vi "Sensor Scaling.vi"(8 "error in":errorcluster) -> (0 "error out":errorcluster, 3 "Output":cluster{"X":dbl[], "Y":dbl[], "Avg point":i16}[](array[cluster]))   [LabVIEW 2015]
uses:
  <vilib>/Analysis/NI_AALPro.lvlib
panel:
  in  "Avg Point":i16=1 min=1 max=500
  out "Offset":dbl format="%0.2f"
  out "Slope":dbl format="%0.2f"
  in  "Unit":string
  in  "Sensor":u16(ring) items=["Load Cell", "LVDT", "LOadcell1", "wq", "load3", "LVDT3", "gggh"]
  in  "Next":bool
  in  "Input Values":dbl[](array[numeric])
  in  "New Calibration":dbl[](array[numeric])
  in  "Sensor Add":bool
  in  "Graph Plot":bool
  in  "Help Button":bool
  in  "Quit":bool
  in  "Save":bool
  out "XY Graph":T1(graph)
  out "error out 2":errorcluster
  out "Numeric":dbl
  out "Old Calibration":dbl[](array[numeric])
  # "Sensor Calibration"
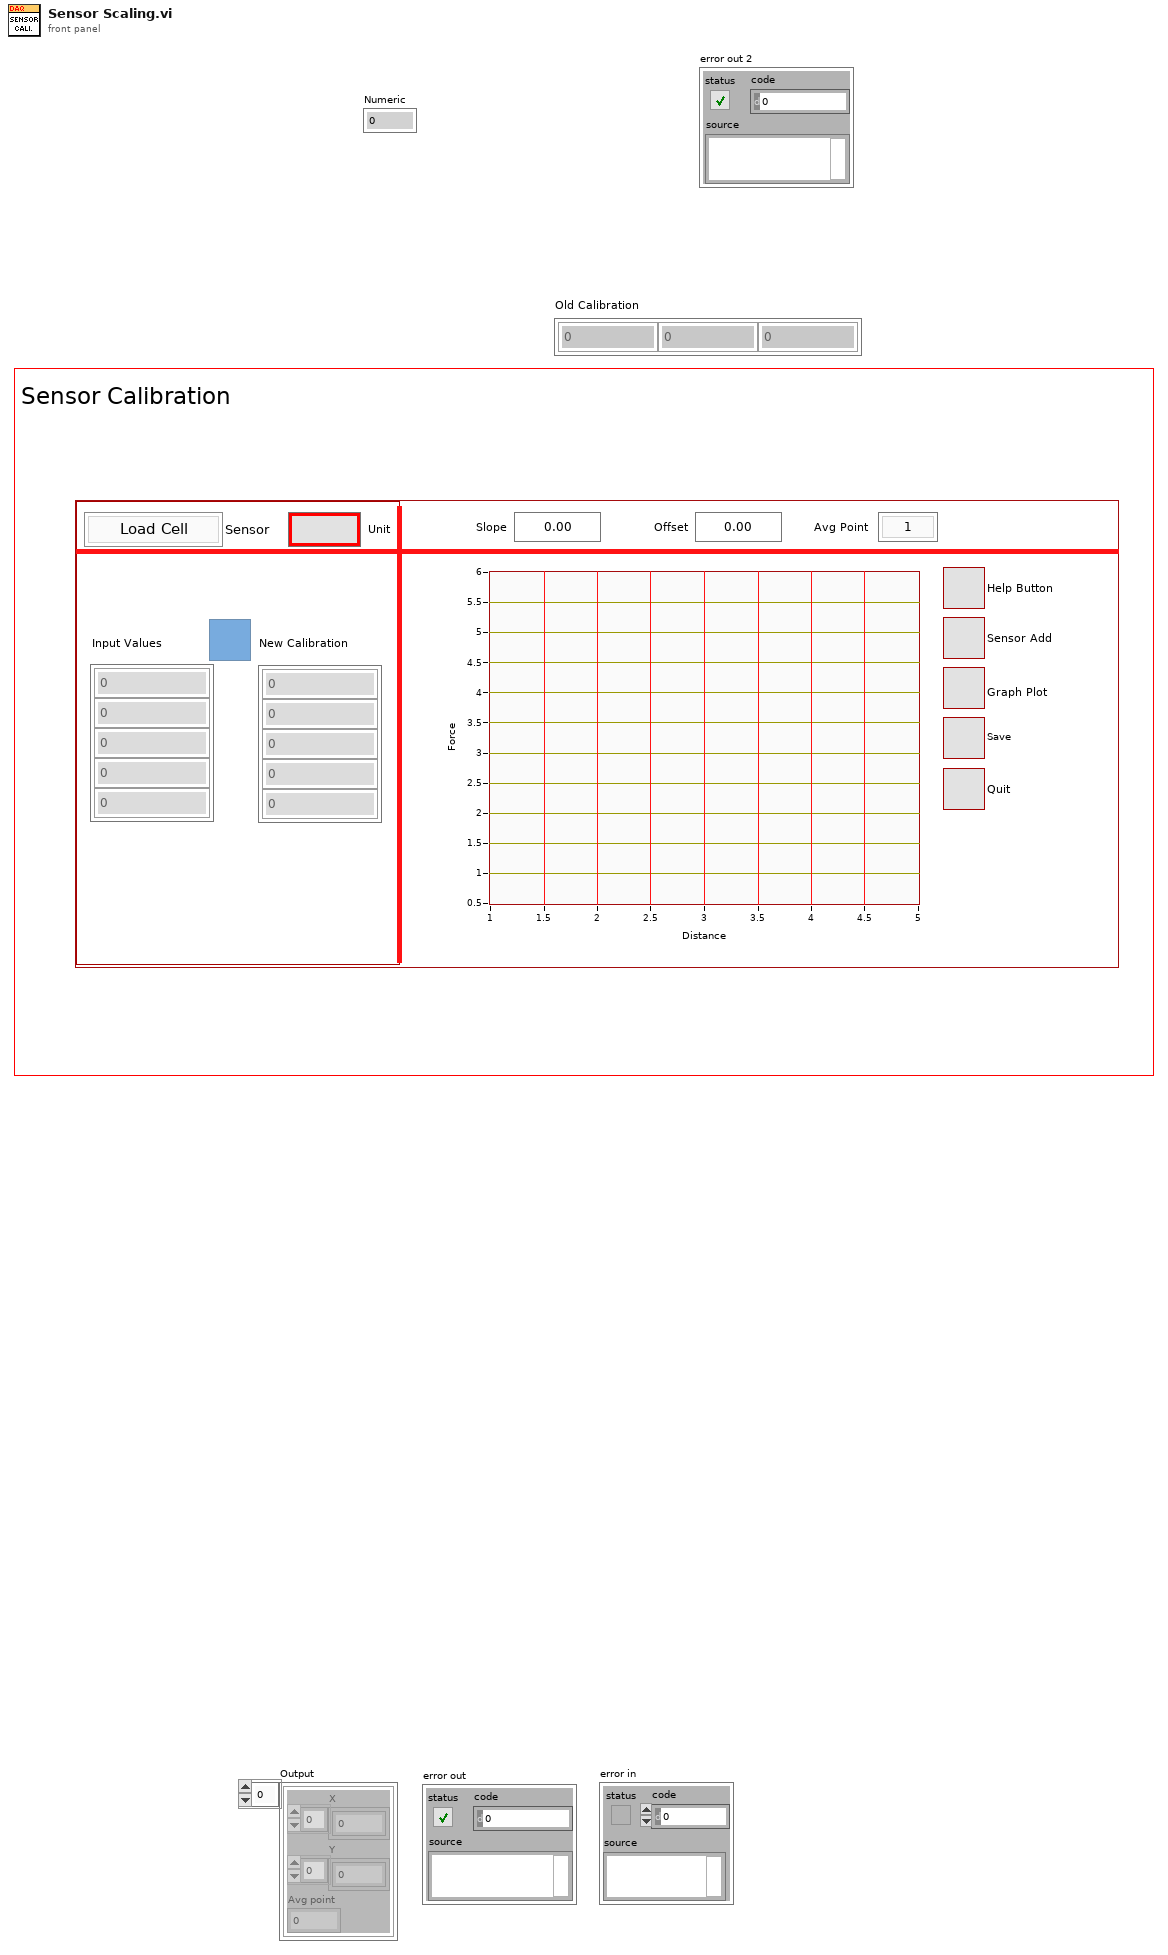
[diagram p1: front panel]
types:
  T1 = cluster{"Input Values":dbl[], "New Calibration":dbl[]}
  T2 = cluster{"XInput":dbl[], "Y New Value":dbl[], "Avg point":i16}[]
  T3 = cluster{"XInput":dbl[], "Y New Value":dbl[], "Avg point":i16}
  T4 = cluster{"Input Values":dbl[], "New Calibration":dbl[], "Sensor":u16}
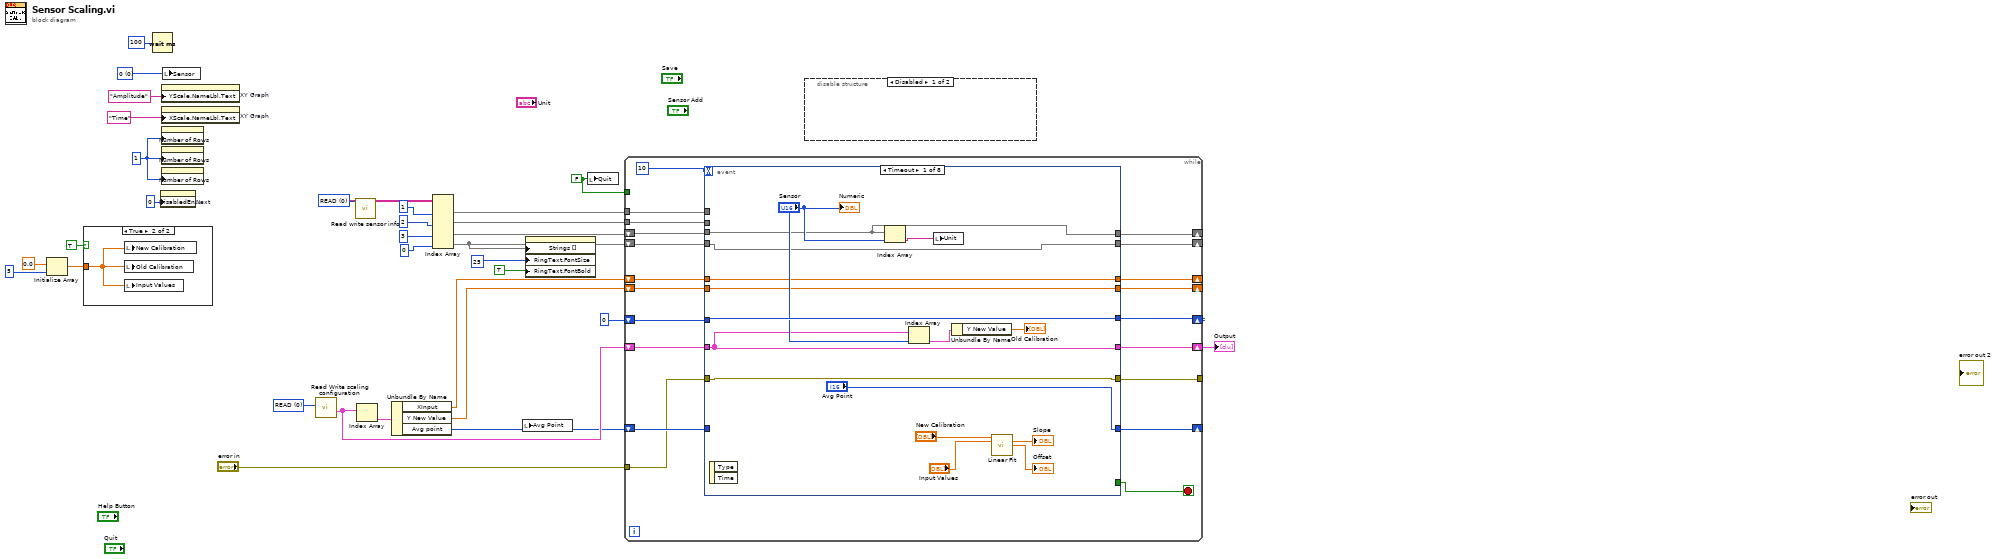
[diagram p0: block diagram]
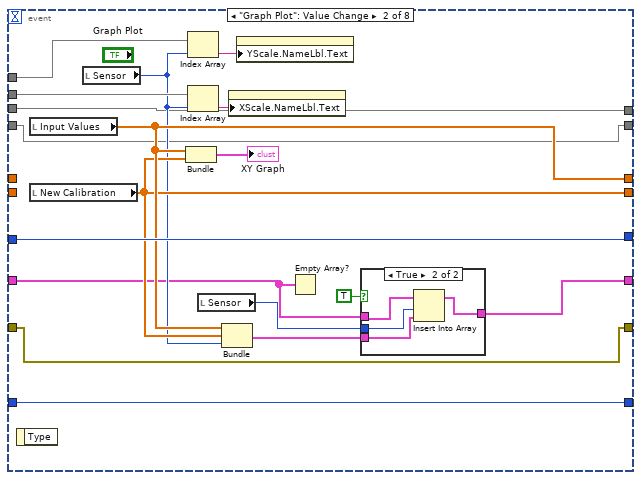
[diagram p4: hidden frame]
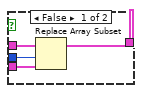
[diagram p5: hidden frame]
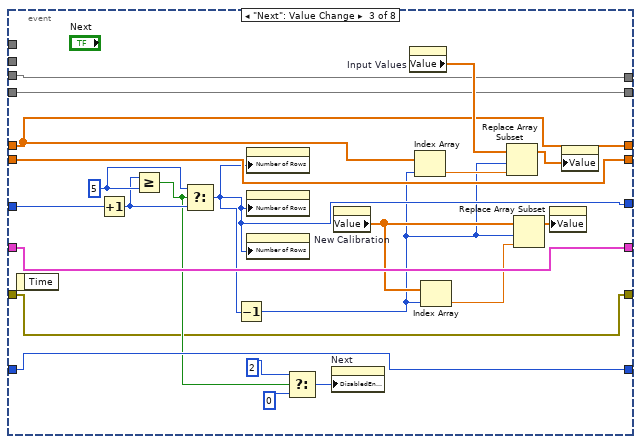
[diagram p6: hidden frame]
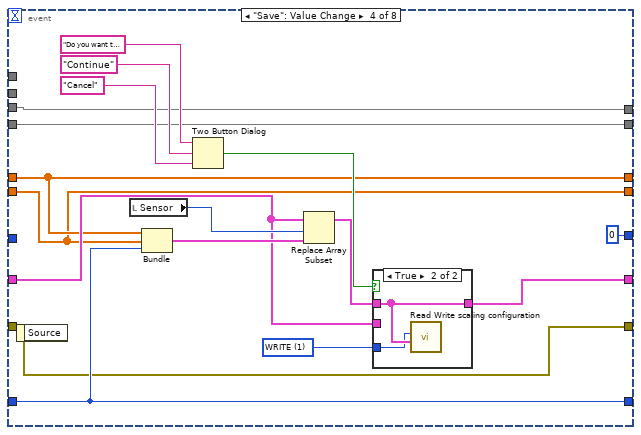
[diagram p7: hidden frame]
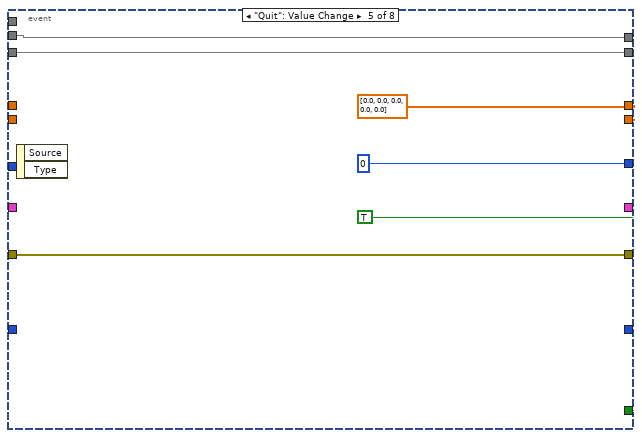
[diagram p9: hidden frame]
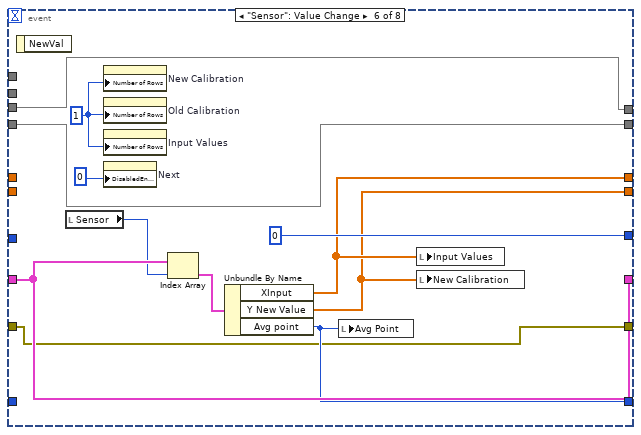
[diagram p10: hidden frame]
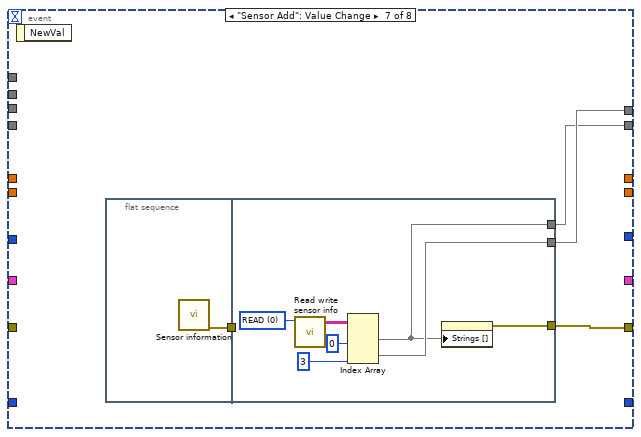
[diagram p11: hidden frame]
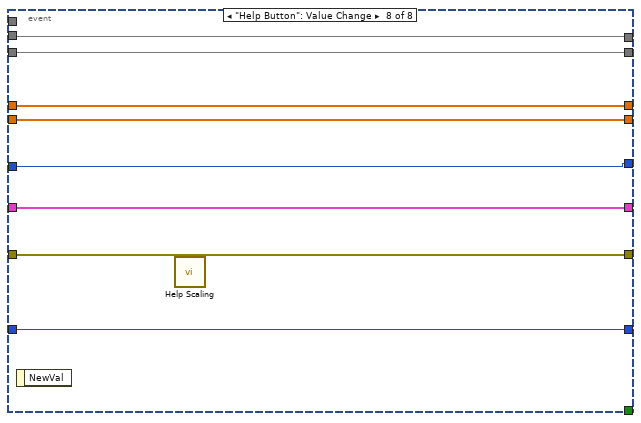
[diagram p12: hidden frame]
diagram:
  w3 = FALSE ("Quit")
  w13 = u16 0 items=["READ", "WRITE"] ("Read/Write")
  w21 = u16 0 items=["READ", "WRITE"] ("Read/Write")
  w9 = u32 1 ("Number of Rows")
  w29 = u16 0 items=["0", "1", "2", "3", "4", "5", "6", "7", "8", "9", "10", "11", "12", "13", "14", "15", "16", "17", "18", "19", "20", "21", "22", "23", "24", "25", "26", "27", "28", "29"] ("Ring")
  n1 = Initialize Array(0.0 ("element"), 5 ("dimension size")) -> (w20:dbl[])
  n2 = case shown="True" TRUE {
    tunnel: w20 -> [_ w33]
    frame False {
    }
    frame True {
      n3 = local write "New Calibration"(w33) -> ()
      n4 = local write "Old Calibration"(w33) -> ()
      n5 = local write "Input Values"(w33) -> ()
    }
  }
  n6 = Wait (ms)(milliseconds to wait=u32 100) -> ()  [unwired: 1 out]
  n7 = property on="Next" class="Bool"("DisabledEnum"=u16 0) -> ()  [unwired: 2 in, 2 out]
  n8 = property on="XY Graph" class="XYGraph (strict)"("YScale.NameLbl.Text"="Amplitude" ("Y Scale.Name Label.Text")) -> ()  [unwired: 2 in, 2 out]
  n9 = property on="XY Graph" class="XYGraph (strict)"("XScale.NameLbl.Text"="Time" ("X Scale.Unit Label.Text")) -> ()  [unwired: 2 in, 2 out]
  n10 = property on="Old Calibration" class="Arr (strict)"("Number of Rows"=w9) -> ()  [unwired: 2 in, 2 out]
  n11 = property on="Input Values" class="Arr (strict)"("Number of Rows"=w9) -> ()  [unwired: 2 in, 2 out]
  n12 = property on="New Calibration" class="Arr (strict)"("Number of Rows"=w9) -> ()  [unwired: 2 in, 2 out]
  n13 = local write "Sensor"(w29) -> ()
  n14 = call "Read Write scaling configuration.vi"("Read/Write"=w21) -> ("Output"=w18:T2)  [unwired: 4 in, 2 out]
  n15 = call "Read write sensor info.vi"("Read/Write"=w13) -> ("Table Control out"=w12:string[][])  [unwired: 9 in, 1 out]
  n16 = Index Array(array=w18) -> (element=w19:T3)  [unwired: 1 in]
  n17 = Unbundle By Name(w19) -> ("XInput"=w7:dbl[], "Y New Value"=w6:dbl[], "Avg point"=w16:i16)
  n18 = Index Array(array=w12, index (col) #1=1 ("disabled index (col)"), index (col) #2=2 ("index (row)"), index (col) #3=3 ("index (row)"), index (col) #4=0 ("index (row)")) -> (element #1=w26:string[], element #2=w25:string[], element #3=w5:string[], element #4=w4:string[])  [unwired: 4 in]
  n19 = local write "Avg Point"(w16) -> ()
  n20 = property on="Sensor" class="Ring (strict)"("Strings []"=w4, "RingText.FontSize"=u32 25 ("Ring Text.Font:Size"), "RingText.FontBold"=TRUE ("Ring Text.Font:Bold")) -> ()  [unwired: 2 in, 2 out]
  n21 = local write "Quit"(w3) -> ()
  n22 = while {
    shift-right: [w51] -> _
    shift-left: i8 0 -> [w52]
    shift-right: [w50] -> _
    shift-left: w6 -> [w49]
    tunnel: w26 -> [w47]
    tunnel: w25 -> [w46]
    shift-right: [w45] -> _
    shift-left: w7 -> [w44]
    shift-right: [w42] -> w15
    shift-left: w18 -> [w43]
    shift-right: [w41] -> _
    shift-left: w16 -> [w40]
    tunnel: [w38] -> _
    tunnel: "error in" -> [w35]
    shift-right: [w37] -> _
    shift-left: w5 -> [w36]
    shift-right: [w34] -> _
    shift-left: w4 -> [w39]
    tunnel: w3 -> [_]
    stop <- w48 stop-if-true
    n23 = event shown="[0] Timeout" {
      selector: _ -> [_ _ _ _ _ _ _ _]
      dyn-events: _ -> [_ _ _ _ _ _ _ _]
      timeout: 10 -> [_ _ _ _ _ _ _ _]
      tunnel: [_ _ _ _ TRUE _ _ _] -> w48
      tunnel: w52 -> [w69 w83 w117 _ _ _ _ w170]
      tunnel: [w69 w83 w107 i8 0 i8 0 i8 0 ("y") _ w170] -> w51
      tunnel: [w63 w77 w113 w122 w141 w147 _ w173] -> w50
      tunnel: w49 -> [w63 _ w113 w122 _ _ _ w173]
      tunnel: w47 -> [_ w87 _ _ _ _ _ _]
      tunnel: w46 -> [_ w86 _ _ _ _ _ _]
      tunnel: w36 -> [w57 w72 w98 w120 w140 w146 _ w175]
      tunnel: [w64 w78 w110 w123 w141 w148 _ w174] -> w45
      tunnel: w44 -> [w64 _ w110 w123 _ _ _ w174]
      tunnel: w43 -> [w65 w74 w114 w125 _ w154 _ w172]
      tunnel: [w65 w75 w114 w129 _ w154 _ w172] -> w42
      tunnel: ["Avg Point" w82 w106 w126 _ w151 _ w171] -> w41
      tunnel: w40 -> [_ w82 w106 w126 _ _ _ w171]
      tunnel: w39 -> [w55 w70 w96 w118 w138 w144 _ w168]
      tunnel: [w56 w71 w97 w119 w139 w145 w158 w169] -> w38
      tunnel: [w57 w72 w98 w120 w140 w146 w157 w175] -> w37
      tunnel: w35 -> [w56 w71 w97 w119 w139 w145 _ w169]
      tunnel: [w55 w70 w96 w118 w138 w144 w156 w168] -> w34
      event Timeout {
        n24 = event-data() -> ()  [unwired: 3 out]
        n25 = Index Array(array=w57, index="Sensor") -> (element=w54:string)
        n26 = Index Array(array=w65, index="Sensor") -> (element=w67:T3)
        n27 = local write "Unit"(w54) -> ()
        n28 = Unbundle By Name(w67) -> ("Y New Value"=→"Old Calibration":dbl[])
        n29 = call <vilib>:"Linear Fit.vi"("Y"="New Calibration", "X"="Input Values") -> ("slope"=→"Slope":dbl, "intercept"=→"Offset":dbl)  [unwired: 9 in, 3 out]
        "Numeric" <- "Sensor"
      }
      event "Graph Plot": Value Change {
        n30 = event-data() -> ()  [unwired: 2 out]
        n31 = local read "Input Values"() -> (w78:dbl[])
        n32 = local read "New Calibration"() -> (w77:dbl[])
        n33 = local read "Sensor"() -> (w76:u16)
        n34 = Bundle("Input Values"=w78, "New Calibration"=w77) -> (→"XY Graph":T1)  [unwired: 1 in]
        n35 = Index Array(array=w87, index=w76) -> (element=w85:string)
        n36 = Index Array(array=w86, index=w76) -> (element=w84:string)
        n37 = local read "Sensor"() -> (w79:u16)
        n38 = Bundle("Input Values"=w78, "New Calibration"=w77, "Sensor"=w76) -> (w80:T4)  [unwired: 1 in]
        n39 = property on="XY Graph" class="XYGraph (strict)"("XScale.NameLbl.Text"=w84) -> ()  [unwired: 2 in, 2 out]
        n40 = property on="XY Graph" class="XYGraph (strict)"("YScale.NameLbl.Text"=w85) -> ()  [unwired: 2 in, 2 out]
        n41 = Empty Array?(array=w74) -> ()  [unwired: 1 out]
        n42 = case shown="True" TRUE {
          tunnel: w80 -> [w91 w93]
          tunnel: w79 -> [w90 w95]
          tunnel: w74 -> [w89 w94]
          tunnel: [w88 w92] -> w75
          frame False {
            n43 = Replace Array Subset(array=w89, new element=w91, index=w90) -> (w88:T2)
          }
          frame True {
            n44 = Insert Into Array(array=w94, index=w95, new element=w93) -> (w92:T2)
          }
        }
      }
      event "Next": Value Change {
        w116 = i8 5 ("y")
        n45 = event-data() -> ()  [unwired: 2 out]
        n46 = Increment(x=w117) -> (x+1=w115:i8)
        n47 = Greater Or Equal?(x=w115, y=w116) -> (x >= y?=w105:bool)
        n48 = Select(t=w116, s=w105, f=w115) -> (s? t:f=w107:i8)
        n49 = Decrement(x=w107) -> (x-1=w100:i8)
        n50 = property on="New Calibration" class="Arr (strict)"("Number of Rows"=w107) -> ()  [unwired: 2 in, 2 out]
        n51 = property on="Old Calibration" class="Arr (strict)"("Number of Rows"=w107) -> ()  [unwired: 2 in, 2 out]
        n52 = property on="Input Values" class="Arr (strict)"("Number of Rows"=w107) -> ()  [unwired: 2 in, 2 out]
        n53 = Select(t=2, s=w105, f=0) -> (s? t:f=w102:i32)
        n54 = property on="Next" class="Bool"("DisabledEnum"=w102) -> ()  [unwired: 2 in, 2 out]
        n55 = property on="New Calibration" class="Arr (strict)"() -> ("Value"=w101:dbl[])  [unwired: 2 in, 2 out]
        n56 = property on="Input Values" class="Arr (strict)"() -> ("Value"=w111:dbl[])  [unwired: 2 in, 2 out]
        n57 = Index Array(array=w110, index=w100) -> (element=w109:dbl)
        n58 = Index Array(array=w101, index=w100) -> (element=w99:dbl)
        n59 = Replace Array Subset(array=w111, new element=w109, index=w100) -> (w112:dbl[])
        n60 = Replace Array Subset(array=w101, new element=w99, index=w100) -> (w108:dbl[])
        n61 = property on="New Calibration" class="Arr (strict)"("Value"=w108) -> ()  [unwired: 2 in, 2 out]
        n62 = property on="Input Values" class="Arr (strict)"("Value"=w112) -> ()  [unwired: 2 in, 2 out]
      }
      event "Save": Value Change {
        w121 = u16 1 items=["READ", "WRITE"] ("Read/Write")
        n63 = event-data() -> ()  [unwired: 2 out]
        n64 = local read "Sensor"() -> (w128:u16)
        n65 = Bundle("XInput"=w123, "Y New Value"=w122, "Avg point"=w126) -> (w127:T3)  [unwired: 1 in]
        n66 = Two Button Dialog(message="Do you want to save new calibration value?", 1:"Cancel" ("T button name (\"OK\")"), 2:"Continue" ("F button name (\"Cancel\")")) -> (T button?=w130:bool)
        n67 = Replace Array Subset(array=w125, new element=w127, index=w128) -> (w124:T2)
        n68 = case shown="True" w130 {
          tunnel: w124 -> [_ w137]
          tunnel: [w135 w137] -> w129
          tunnel: w125 -> [w135 _]
          tunnel: w121 -> [_ w136]
          frame False {
          }
          frame True {
            n69 = call "Read Write scaling configuration.vi"("Input"=w137, "Read/Write"=w136) -> ()  [unwired: 3 in, 3 out]
          }
        }
      }
      event "Quit": Value Change {
        w141 = dbl[] [0.0, 0.0, 0.0, 0.0, 0.0]
        n70 = event-data() -> ()  [unwired: 3 out]
      }
      event "Sensor": Value Change {
        w149 = u32 1 ("Number of Rows")
        n71 = event-data() -> ()  [unwired: 2 out]
        n72 = local read "Sensor"() -> (w152:u16)
        n73 = property on="New Calibration" class="Arr (strict)"("Number of Rows"=w149) -> ()  [unwired: 2 in, 2 out]
        n74 = property on="Old Calibration" class="Arr (strict)"("Number of Rows"=w149) -> ()  [unwired: 2 in, 2 out]
        n75 = property on="Input Values" class="Arr (strict)"("Number of Rows"=w149) -> ()  [unwired: 2 in, 2 out]
        n76 = property on="Next" class="Bool"("DisabledEnum"=0) -> ()  [unwired: 2 in, 2 out]
        n77 = Index Array(array=w154, index=w152) -> (element=w155:T3)
        n78 = Unbundle By Name(w155) -> ("XInput"=w148:dbl[], "Y New Value"=w147:dbl[], "Avg point"=w151:i16)
        n79 = local write "Avg Point"(w151) -> ()
        n80 = local write "Input Values"(w148) -> ()
        n81 = local write "New Calibration"(w147) -> ()
      }
      event "Sensor Add": Value Change {
        n82 = event-data() -> ()  [unwired: 2 out]
        n83 = flat-sequence {
          tunnel: [w160] -> w159
          tunnel: w159 -> [_]
          tunnel: [w164] -> w158
          tunnel: [w162] -> w157
          tunnel: [w161] -> w156
          frame #0 {
            n84 = call "Sensor information.vi"() -> ("error in (no error) 2"=w160:errorcluster)  [unwired: 11 in]
          }
          frame #1 {
            w167 = u16 0 items=["READ", "WRITE"] ("Read/Write")
            n85 = call "Read write sensor info.vi"("Read/Write"=w167) -> ("Table Control out"=w166:string[][])  [unwired: 9 in, 1 out]
            n86 = Index Array(array=w166, index (col) #1=0 ("disabled index (col)"), index (col) #2=3 ("index (col)")) -> (element #1=w161:string[], element #2=w162:string[])  [unwired: 2 in]
            n87 = property on="Sensor" class="Ring (strict)"("Strings []"=w161) -> (error out=w164:errorcluster)  [unwired: 2 in, 1 out]
          }
        }
      }
      event "Help Button": Value Change {
        n88 = event-data() -> ()  [unwired: 2 out]
        n89 = call "Help Scaling.vi"() -> ()  [unwired: 12 in]
      }
    }
  }
  "Output" <- w15
  n90 = disable-structure shown="Disabled" {
    frame Disabled {
    }
    frame Enabled {
    }
  }
